vi "6509 Control Outputs AUX.vi"(1 "device name":tag="Dev1", 2 "error in (no error)":errorcluster, 3 "Enable Output":bool, 4 "Enum":T1(ring)) -> (0 "error out":errorcluster)   [LabVIEW 2014]
panel:
  in  "data":bool[](array[boolean])
  # "Pos 4"
  # "pos 5"
  # "Pos 10"
  # "Pos 11"
  # "Pos 12"
  # "Pos 13"
  # "Pos 14"
  # "Pos 15"
  # "Pos 7"
  # "Pos 0"
  # "Pos 1"
  # "Pos 2"
  # "Pos 3"
  # "Pos 6"
  # "Pos 8"
  # "Pos 9"
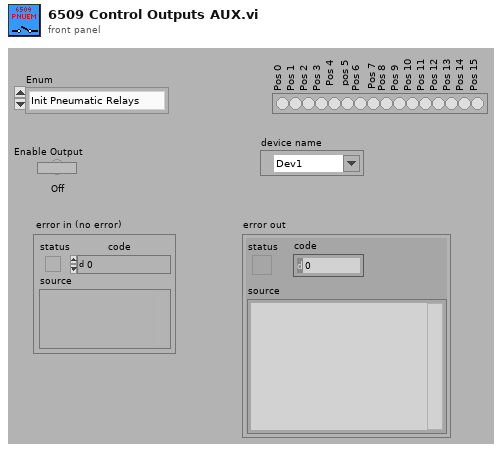
[diagram p1: front panel]
types:
  T1 = enum16{"Init Pneumatic Relays", "P2.0", "P2.1", "P2.2", "P2.3", "P2.4", "P2.5"}
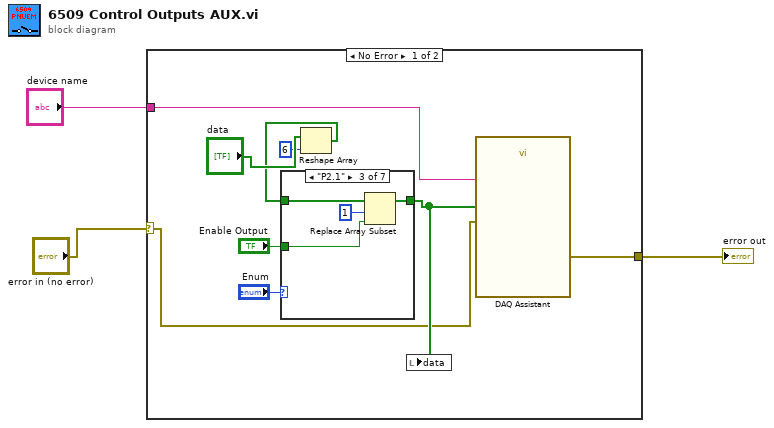
[diagram p0: block diagram]
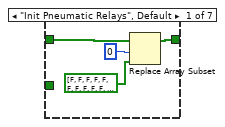
[diagram p2: hidden frame]
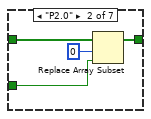
[diagram p3: hidden frame]
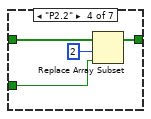
[diagram p4: hidden frame]
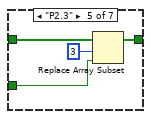
[diagram p5: hidden frame]
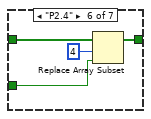
[diagram p6: hidden frame]
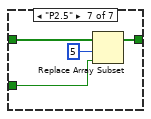
[diagram p7: hidden frame]
diagram:
  n1 = case shown="No Error" "error in (no error)" {
    selector: "error in (no error)" -> [w5 w41]
    tunnel: [w11 w41] -> w3
    tunnel: "device name" -> [w4 _]
    frame No Error {
      n2 = Reshape Array("data", 6 ("dimension size")) -> (w7:bool[])
      n3 = case shown="\"P2.1\"" "Enum" {
        tunnel: "Enable Output" -> [_ w18 w22 w26 w30 w34 w38]
        tunnel: w7 -> [w16 w19 w23 w27 w31 w35 w39]
        tunnel: [w14 w17 w21 w25 w29 w33 w37] -> w6
        frame "Init Pneumatic Relays", Default {
          n4 = Replace Array Subset(array=w16, new element=bool[] [FALSE, FALSE, FALSE, FALSE, FALSE, FALSE, FALSE, FALSE, FALSE, FALSE, FALSE, FALSE, FALSE, FALSE, FALSE, FALSE, FALSE, FALSE, FALSE, FALSE, FALSE, FALSE, FALSE, FALSE] ("data 2"), index=0) -> (w14:bool[])
        }
        frame "P2.0" {
          n5 = Replace Array Subset(array=w19, new element=w18, index=0) -> (w17:bool[])
        }
        frame "P2.1" {
          n6 = Replace Array Subset(array=w23, new element=w22, index=1) -> (w21:bool[])
        }
        frame "P2.2" {
          n7 = Replace Array Subset(array=w27, new element=w26, index=2) -> (w25:bool[])
        }
        frame "P2.3" {
          n8 = Replace Array Subset(array=w31, new element=w30, index=3) -> (w29:bool[])
        }
        frame "P2.4" {
          n9 = Replace Array Subset(array=w35, new element=w34, index=4) -> (w33:bool[])
        }
        frame "P2.5" {
          n10 = Replace Array Subset(array=w39, new element=w38, index=5) -> (w37:bool[])
        }
      }
      n11 = local write "data"(w6) -> ()
      n12 = call "DAQ Assistant"("data"=w6, "error in"=w5, "device name"=w4) -> ("error out"=w11:errorcluster)  [unwired: 15 in, 1 out]
    }
    frame Error {
    }
  }
  "error out" <- w3
